vi "single tp string.vi"(9 "value in":string[](array[string]), 11 "oringnal defult tp data":string="[Pause Message test]\nExt.Name =;\nOutput string =;#") -> (2 "new single tp data out":string="[Pause Message test]\nExt.Name =;\nOutput string =;#")   [LabVIEW 2018]
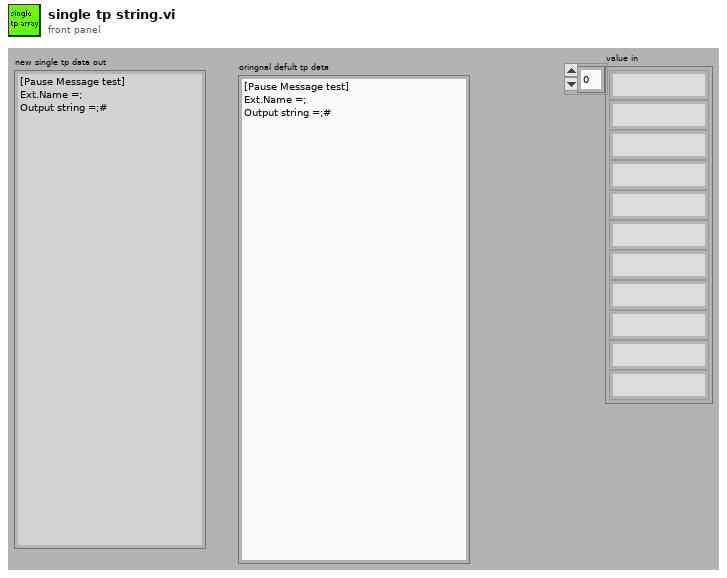
[diagram p1: front panel]
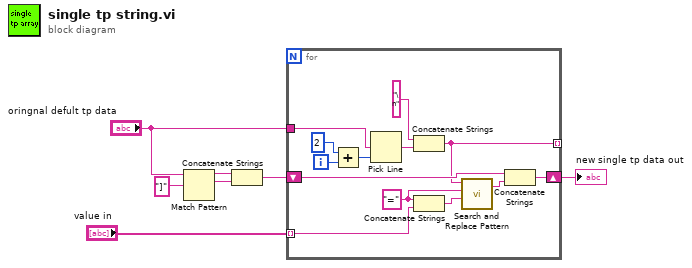
[diagram p0: block diagram]
diagram:
  n1 = Match Pattern(string="oringnal defult tp data", regular expression="]" ("正则表达式")) -> (before substring=w6:string, match substring=w5:string)  [unwired: 3 out]
  n2 = Concatenate Strings(w6, w5) -> (w4:string)
  n3 = for {
    tunnel: "oringnal defult tp data" -> [w10]
    shift-right: [w20] -> w1
    shift-left: w4 -> [w19]
    tunnel: "value in" -> [w14] mode=indexing
    tunnel: [w9] -> _ mode=indexing
    i -> [w18]
    w13 = "=" ("regular expression (\"\")")
    n4 = Add(x=2, y=w18) -> (x+y=w17:i32)
    n5 = Pick Line(multi-line string=w10, line index=w17) -> (output string=w16:string)  [unwired: 1 out]
    n6 = Concatenate Strings("\n" ("字符串"), w16) -> (w9:string)
    n7 = Concatenate Strings(w13, w14) -> (w12:string)
    n8 = call <vilib>:"Search and Replace Pattern.vi"("string"=w9, "regular expression (\"\")"=w13, "replace string (\"\")"=w12) -> ("result string"=w11:string)  [unwired: 3 out]
    n9 = Concatenate Strings(w19, w11) -> (w20:string)
  }
  "new single tp data out" <- w1
